vi "空载判定.vi"(0 "曲线引用":refnum<vi>, 1 "曲线":u32, 2 "曲线判定条件":T1, 3 "错误输入":errorcluster) -> (7 "曲线引用输出":refnum<vi>, 8 "判定结果":cluster{"合格？":bool, "判定结果":string[][]}, 10 "错误输出":errorcluster)   [LabVIEW 2018]
uses:
  <userlib>/_MGI/1D Array/MGI Average/MGI Average (DBL[]).vi
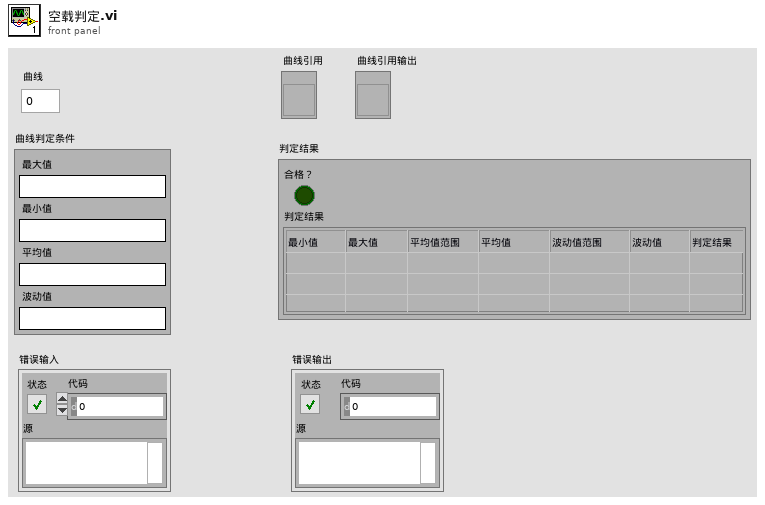
[diagram p1: front panel]
types:
  T1 = cluster{"最大值":string, "最小值":string, "平均值":string, "波动值":string}
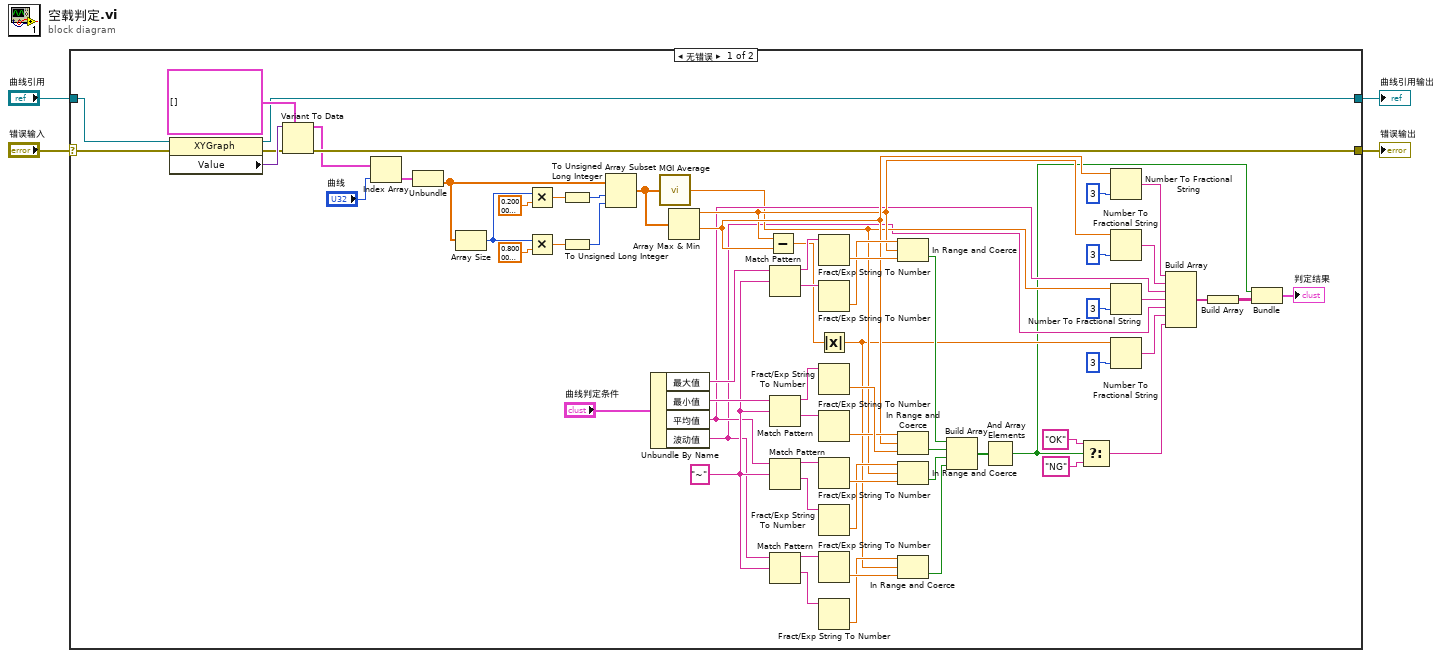
[diagram p0: block diagram]
diagram:
  n1 = case shown="无错误" "错误输入" {
    selector: "错误输入" -> [w68 w72]
    tunnel: [w15 w72] -> w3
    tunnel: "曲线引用" -> [w18 w71]
    tunnel: [w17 w71] -> w1
    frame No Error {
      w64 = "~" ("正则表达式")
      n2 = property class="XYGraph"(reference=w18, error in=w68) -> (reference out=w17:refnum<vi>, error out=w16:errorcluster, "Value"=w70:variant)
      n3 = Variant To Data(error in=w16, type=cluster{dbl[], dbl[]}[] [], Variant=w70) -> (data=w7:cluster{dbl[], dbl[]}[], error out=w15:errorcluster)
      n4 = Index Array(array=w7, index="曲线") -> (element=w63:cluster{dbl[], dbl[]})
      n5 = Unbundle(w63) -> (w6:dbl[])  [unwired: 1 out]
      n6 = Array Size(array=w6) -> (size(s)=w11:i32)
      n7 = Multiply(x=w11, y=sgl 0.2) -> (x*y=w10:sgl)
      n8 = Multiply(x=w11, y=sgl 0.8) -> (x*y=w12:sgl)
      n9 = To Unsigned Long Integer(number=w10) -> (unsigned 32bit integer=w13:u32)
      n10 = To Unsigned Long Integer(number=w12) -> (unsigned 32bit integer=w14:u32)
      n11 = Array Subset(array=w6, index=w13, length=w14) -> (w5:dbl[])
      n12 = Unbundle By Name("曲线判定条件") -> ("最大值"=w66:string, "最小值"=w65:string, "平均值"=w35:string, "波动值"=w29:string)
      n13 = call-poly <userlib>:"MGI Average.vi"("Double[]"=w5) -> ("Average"=w31:dbl)  [unwired: 1 in]
      n14 = Array Max & Min(array=w5) -> (max value=w38:dbl, min value=w40:dbl)  [unwired: 2 out]
      n15 = Subtract(x=w38, y=w40) -> (x-y=w45:dbl)
      n16 = Match Pattern(string=w66, regular expression=w64) -> (before substring=w61:string, after substring=w60:string)  [unwired: 1 in, 2 out]
      n17 = Match Pattern(string=w65, regular expression=w64) -> (before substring=w59:string, after substring=w58:string)  [unwired: 1 in, 2 out]
      n18 = Match Pattern(string=w35, regular expression=w64) -> (before substring=w57:string, after substring=w56:string)  [unwired: 1 in, 2 out]
      n19 = Match Pattern(string=w29, regular expression=w64) -> (before substring=w55:string, after substring=w54:string)  [unwired: 1 in, 2 out]
      n20 = Fract/Exp String To Number(string=w61) -> (number=w53:dbl)  [unwired: 3 in, 1 out]
      n21 = Fract/Exp String To Number(string=w60) -> (number=w52:dbl)  [unwired: 3 in, 1 out]
      n22 = Absolute Value(x=w45) -> (abs(x)=w28:dbl)
      n23 = Fract/Exp String To Number(string=w59) -> (number=w51:dbl)  [unwired: 3 in, 1 out]
      n24 = Fract/Exp String To Number(string=w58) -> (number=w50:dbl)  [unwired: 3 in, 1 out]
      n25 = Fract/Exp String To Number(string=w57) -> (number=w49:dbl)  [unwired: 3 in, 1 out]
      n26 = Fract/Exp String To Number(string=w56) -> (number=w48:dbl)  [unwired: 3 in, 1 out]
      n27 = Fract/Exp String To Number(string=w55) -> (number=w47:dbl)  [unwired: 3 in, 1 out]
      n28 = Fract/Exp String To Number(string=w54) -> (number=w46:dbl)  [unwired: 3 in, 1 out]
      n29 = In Range and Coerce(upper limit=w52, x=w38, lower limit=w53) -> (In Range?=w44:bool)  [unwired: 1 out]
      n30 = In Range and Coerce(upper limit=w50, x=w40, lower limit=w51) -> (In Range?=w43:bool)  [unwired: 1 out]
      n31 = In Range and Coerce(upper limit=w48, x=w31, lower limit=w49) -> (In Range?=w42:bool)  [unwired: 1 out]
      n32 = In Range and Coerce(upper limit=w46, x=w28, lower limit=w47) -> (In Range?=w41:bool)  [unwired: 1 out]
      n33 = Build Array(w44, w43, w42, w41) -> (w26:bool[])
      n34 = And Array Elements(Boolean array=w26) -> (logical AND=w22:bool)
      n35 = Select(t="OK", s=w22, f="NG") -> (s? t:f=w23:string)
      n36 = Number To Fractional String(number=w40, precision (6)=i16 3 ("精度(6)")) -> (F-format string=w37:string)  [unwired: 2 in]
      n37 = Number To Fractional String(number=w38, precision (6)=i16 3 ("精度(6)")) -> (F-format string=w36:string)  [unwired: 2 in]
      n38 = Number To Fractional String(number=w31, precision (6)=i16 3 ("精度(6)")) -> (F-format string=w30:string)  [unwired: 2 in]
      n39 = Number To Fractional String(number=w28, precision (6)=i16 3 ("精度(6)")) -> (F-format string=w27:string)  [unwired: 2 in]
      n40 = Build Array(w37, w36, w35, w30, w29, w27, w23) -> (w20:string[])
      n41 = Build Array(w20) -> (w19:string[][])
      n42 = Bundle(w22, w19) -> (→"判定结果":cluster{bool, string[][]})  [unwired: 1 in]
    }
    frame Error {
    }
  }
  "错误输出" <- w3
  "曲线引用输出" <- w1
